vi "Convert Array to IMPARAMS.vi"(2 "Array":u32[](array[numeric])) -> (16 "IMPARAMS":T1)   [LabVIEW 2013, in "VRI.lvlib"]
uses:
  VRI.lvlib
  _Type Defs/PHCon IMPARAMS.ctl
  _Type Defs/PhInt WBGAIN.ctl
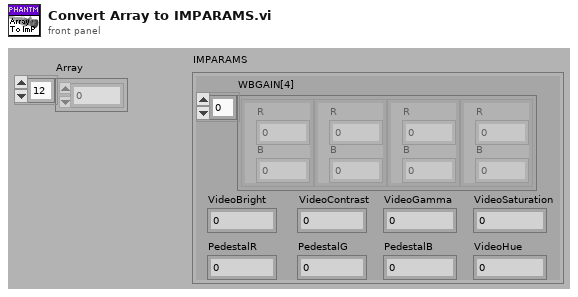
[diagram p1: front panel]
types:
  T1 = typedef "VRI.lvlib/PHCon IMPARAMS.ctl" = cluster{"WBGAIN[4]":T2[], "VideoBright":i32, "VideoContrast":i32, "VideoGamma":sgl, "VideoSaturation":i32, "PedestalR":i32, "PedestalG":i32, "PedestalB":i32, "VideoHue":i32}
  T2 = typedef "VRI.lvlib/PhInt WBGAIN.ctl" = cluster{"R":sgl, "B":sgl}
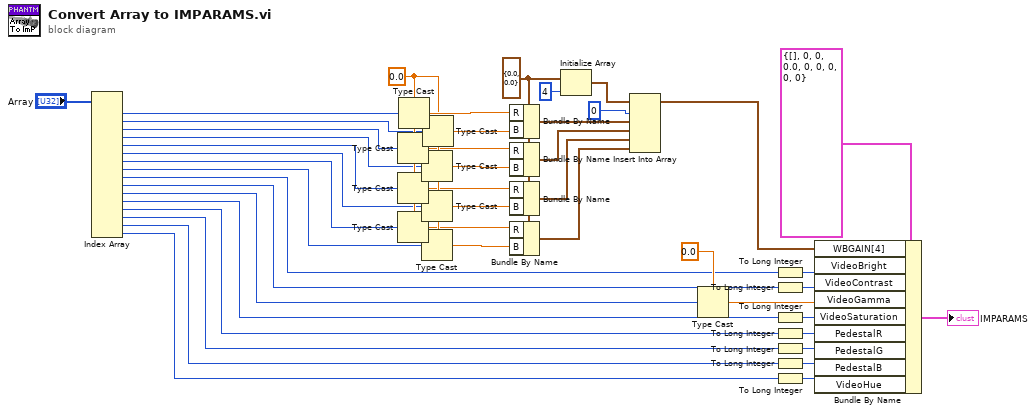
[diagram p0: block diagram]
diagram:
  w14 = sgl 0.0
  w44 = T2 {"R"=0.0, "B"=0.0} ("WBGAIN")
  n1 = Index Array(array="Array") -> (element #1=w24:u32, element #2=w7:u32, element #3=w6:u32, element #4=w5:u32, element #5=w4:u32, element #6=w3:u32, element #7=w2:u32, element #8=w1:u32, element #9=w23:u32, element #10=w22:u32, element #11=w21:u32, element #12=w20:u32, element #13=w19:u32, element #14=w18:u32, element #15=w17:u32, element #16=w16:u32)  [unwired: 16 in]
  n2 = Type Cast(type=w14, x=w6) -> (*(type *) &x=w13:sgl)
  n3 = Type Cast(type=w14, x=w4) -> (*(type *) &x=w11:sgl)
  n4 = Type Cast(type=w14, x=w2) -> (*(type *) &x=w9:sgl)
  n5 = Type Cast(type=w14, x=w24) -> (*(type *) &x=w27:sgl)
  n6 = Type Cast(type=w14, x=w5) -> (*(type *) &x=w12:sgl)
  n7 = Type Cast(type=w14, x=w3) -> (*(type *) &x=w10:sgl)
  n8 = Type Cast(type=w14, x=w1) -> (*(type *) &x=w8:sgl)
  n9 = Type Cast(type=w14, x=w7) -> (*(type *) &x=w15:sgl)
  n10 = Bundle By Name(cluster=w44, "R"=w27, "B"=w15) -> (w41:T2)
  n11 = Bundle By Name(cluster=w44, "R"=w13, "B"=w12) -> (w40:T2)
  n12 = Bundle By Name(cluster=w44, "R"=w11, "B"=w10) -> (w39:T2)
  n13 = Bundle By Name(cluster=w44, "R"=w9, "B"=w8) -> (w38:T2)
  n14 = Initialize Array(w44, 4 ("dimension size")) -> (w42:T2[])
  n15 = Insert Into Array(array=w42, index=0, new element #1=w41, new element #2=w40, new element #3=w39, new element #4=w38) -> (w37:T2[])
  n16 = Type Cast(type=sgl 0.0, x=w21) -> (*(type *) &x=w26:sgl)
  n17 = To Long Integer(number=w23) -> (32bit integer=w36:i32)
  n18 = To Long Integer(number=w22) -> (32bit integer=w35:i32)
  n19 = To Long Integer(number=w20) -> (32bit integer=w34:i32)
  n20 = To Long Integer(number=w19) -> (32bit integer=w33:i32)
  n21 = To Long Integer(number=w18) -> (32bit integer=w32:i32)
  n22 = To Long Integer(number=w17) -> (32bit integer=w31:i32)
  n23 = To Long Integer(number=w16) -> (32bit integer=w30:i32)
  n24 = Bundle By Name(cluster=T1 {"WBGAIN[4]"=[], "VideoBright"=0, "VideoContrast"=0, "VideoGamma"=0.0, "VideoSaturation"=0, "PedestalR"=0, "PedestalG"=0, "PedestalB"=0, "VideoHue"=0} ("IMPARAMS"), "WBGAIN[4]"=w37, "VideoBright"=w36, "VideoContrast"=w35, "VideoGamma"=w26, "VideoSaturation"=w34, "PedestalR"=w33, "PedestalG"=w32, "PedestalB"=w31, "VideoHue"=w30) -> (→"IMPARAMS":T1)
